vi "stop2.vi"(8 "error in (no error)":errorcluster, 10 "stop":bool, 11 "WinX32Camera in":refnum<class "WinX32Camera.lvclass">) -> (0 "error out":errorcluster, 1 "imageSaved":bool, 2 "stopped?":bool, 3 "WinX32Camera out":refnum<class "WinX32Camera.lvclass">)   [LabVIEW 2011, in "WinX32Camera.lvclass"]
uses:
  WinX32Camera.lvclass
  WinX32Camera.lvclass/WinX32Camera.ctl
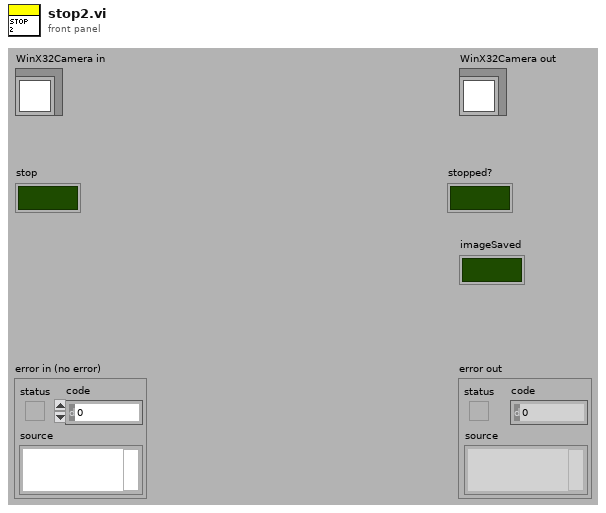
[diagram p1: front panel]
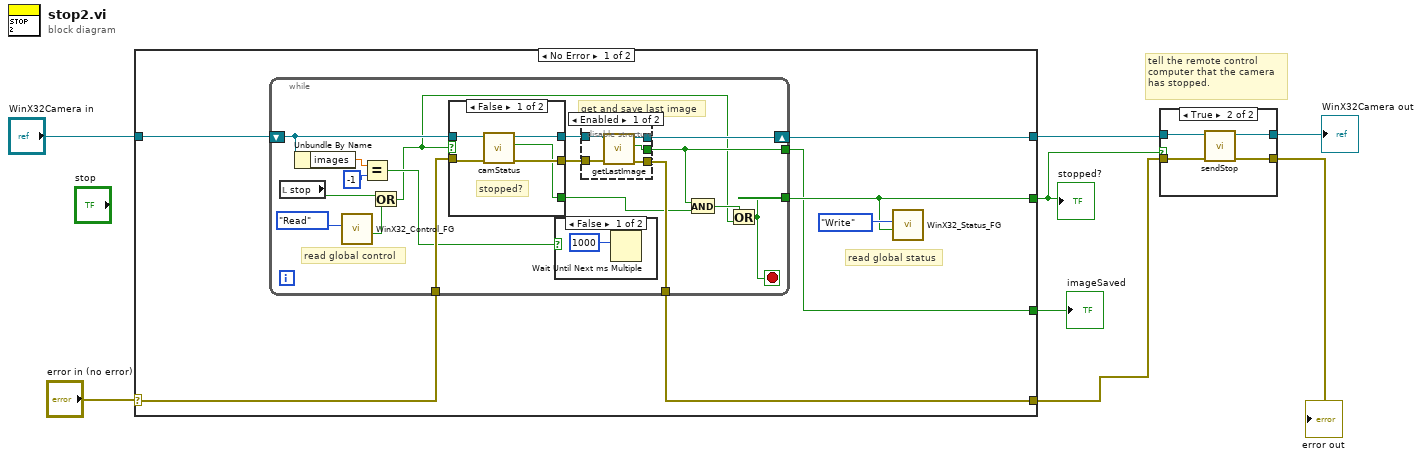
[diagram p0: block diagram]
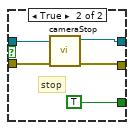
[diagram p5: hidden frame]
diagram:
  # "tell the remote control\ncomputer that the camera\nhas stopped."
  n1 = case shown="No Error" "error in (no error)" {
    selector: "error in (no error)" -> [w14 w52]
    tunnel: [w13 w52] -> w5
    tunnel: [w15 w51] -> w6
    tunnel: "WinX32Camera in" -> [w10 w51]
    tunnel: [w11 _] -> w2
    tunnel: [w9 _] -> w1
    frame No Error {
      # "read global status"
      n2 = while {
        tunnel: w14 -> [w29]
        tunnel: [w16] -> w11
        tunnel: [w28] -> w13
        shift-right: [w30] -> w15
        shift-left: w10 -> [w24]
        tunnel: [w19] -> w9
        stop <- w16 stop-if-true
        # "read global control"
        # "get and save last image"
        n3 = local read "stop"() -> (w26:bool)
        n4 = Unbundle By Name(w24) -> ("images"=w23:dbl)
        n5 = call "WinX32_Control_FG.vi"("Action"=enum16{"Write", "Read"}."Read") -> ("stopped"=w25:bool)  [unwired: 10 in]
        n6 = Equal?(x=w23, y=-1) -> (x = y?=w21:bool)
        n7 = Or(x=w26, y=w25) -> (x .or. y?=w17:bool)
        n8 = case shown="False" w17 {
          tunnel: [w45 w49] -> w32
          tunnel: [w44 w48] -> w31
          tunnel: w24 -> [w43 w50]
          tunnel: w29 -> [w41 w47]
          tunnel: [w42 TRUE] -> w20
          frame False {
            # "stopped?"
            n9 = call "camStatus.vi"("error in (no error)"=w41, "WinX32Camera in"=w43) -> ("error out"=w44:errorcluster, "stopped?"=w42:bool, "WinX32Camera out"=w45:refnum<class "WinX32Camera.lvclass">)  [unwired: 7 in]
          }
          frame True {
            # "stop"
            n10 = call "cameraStop.vi"("error in (no error)"=w47, "WinX32Camera in"=w50) -> ("error out"=w48:errorcluster, "WinX32Camera out"=w49:refnum<class "WinX32Camera.lvclass">)  [unwired: 8 in]
          }
        }
        n11 = case shown="False" w21 {
          frame False {
            n12 = Wait Until Next ms Multiple(millisecond multiple=1000) -> ()  [unwired: 1 out]
          }
          frame True {
          }
        }
        n13 = disable-structure shown="Enabled" {
          disable-tunnel: w32 -> [w38 w39]
          disable-tunnel: w31 -> [w37 w40]
          disable-tunnel: [w36 w39] -> w30
          disable-tunnel: [w35 w40] -> w28
          disable-tunnel: [w34 _] -> w19
          frame Enabled {
            n14 = call "getLastImage.vi"("error in (no error)"=w37, "WinX32Camera in"=w38) -> ("error out"=w35:errorcluster, "All images read"=w34:bool, "WinX32Camera out"=w36:refnum<class "WinX32Camera.lvclass">)  [unwired: 7 in]
          }
          frame Disabled {
          }
        }
        n15 = And(x=w19, y=w20) -> (x .and. y?=w18:bool)
        n16 = Or(x=w18, y=w17) -> (x .or. y?=w16:bool)
      }
      n17 = call "WinX32_Status_FG.vi"("stop"=w11, "Action"=enum16{"Write", "Read"}."Write") -> ()  [unwired: 9 in, 1 out]
    }
    frame Error {
    }
  }
  "stopped?" <- w2
  "imageSaved" <- w1
  n18 = case shown="True" w2 {
    tunnel: w6 -> [w54 w58]
    tunnel: [w54 w57] -> w4
    tunnel: w5 -> [w53 w56]
    tunnel: [w53 w55] -> w3
    frame False {
    }
    frame True {
      n19 = call "sendStop.vi"("error in (no error)"=w56, "WinX32Camera in"=w58) -> ("error out"=w55:errorcluster, "WinX32Camera out"=w57:refnum<class "WinX32Camera.lvclass">)  [unwired: 8 in]
    }
  }
  "error out" <- w3
  "WinX32Camera out" <- w4
